vi "Handle.vi"(8 "error in (no error)":errorcluster, 10 "Error In":errorcluster, 11 "ErrorHandler(Handler) in":refnum<class "ErrorHandler(Handler).lvclass">) -> (0 "error out":errorcluster, 2 "handled?":bool, 3 "ErrorHandler(Handler) out":refnum<class "ErrorHandler(Handler).lvclass">)   [LabVIEW 2014, in "Chain Of Responsibility Pattern.lvlib" / "ErrorHandler(Handler).lvclass"]
uses:
  ErrorHandler(Handler).lvclass
  ErrorHandler(Handler).lvclass/ErrorHandler(Handler).ctl
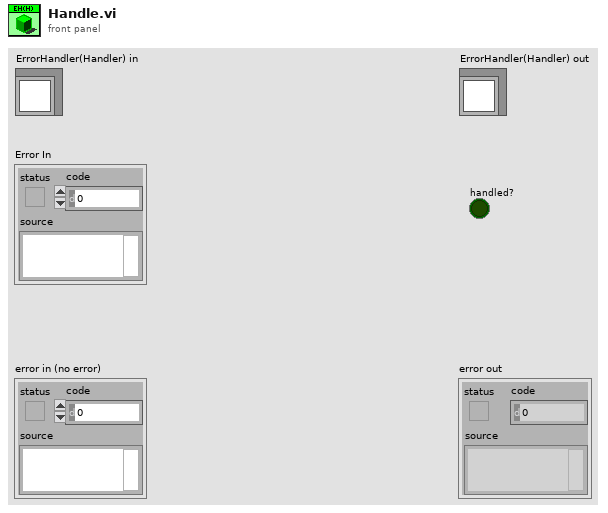
[diagram p1: front panel]
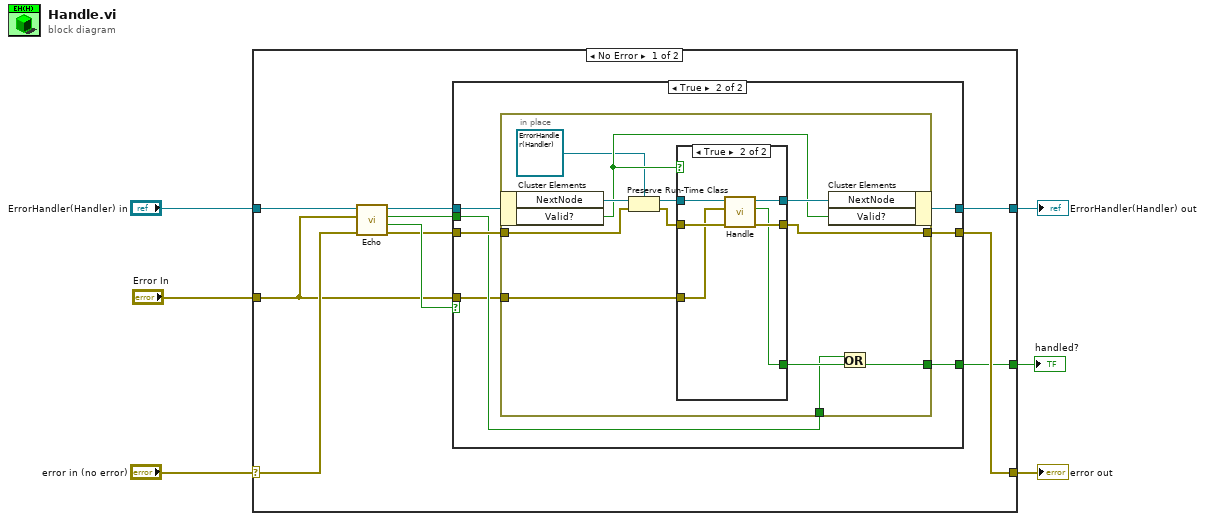
[diagram p0: block diagram]
diagram:
  n1 = case shown="No Error" "error in (no error)" {
    selector: "error in (no error)" -> [w15 w48]
    tunnel: [w10 w48] -> w5
    tunnel: [w11 w47] -> w3
    tunnel: "ErrorHandler(Handler) in" -> [w16 w47]
    tunnel: "Error In" -> [w7 _]
    tunnel: [w8 _] -> w1
    frame No Error {
      n2 = call-dynamic "Echo.vi"("error in (no error)"=w15, "Error In"=w7, "HandlerCore in"=w16) -> ("error out"=w12:errorcluster, "Still Pass?"=w14:bool, "handled?"=w9:bool, "HandlerCore out"=w13:refnum<class "ErrorHandler(Handler).lvclass">)  [unwired: 5 in]
      n3 = case shown="True" w14 {
        tunnel: w13 -> [w19 w25]
        tunnel: w12 -> [w18 w26]
        tunnel: [w19 w24] -> w11
        tunnel: [w18 w23] -> w10
        tunnel: w9 -> [w17 w21]
        tunnel: [w17 w22] -> w8
        tunnel: w7 -> [_ w20]
        frame False {
        }
        frame True {
          n4 = in-place {
            in-place-border: w26 -> [w38]
            in-place-border: [w32] -> w23
            in-place-border: [w29] -> w22
            in-place-border: w21 -> [w28]
            in-place-border: w20 -> [w27]
            n5 = in-place-cluster #1(w25) -> ("NextNode"=w36:refnum<class "HandlerCore.lvclass">, "Valid?"=w33:bool)
            n6 = Preserve Run-Time Class(object in=w36, error in=w38, 2:refnum<class "ErrorHandler(Handler).lvclass"> refnum ("ErrorHandler(Handler)")) -> (object out=w37:refnum<class "ErrorHandler(Handler).lvclass">, error out=w35:errorcluster)
            n7 = case shown="True" w33 {
              tunnel: w37 -> [w40 w46]
              tunnel: w35 -> [w39 w44]
              tunnel: [w40 w45] -> w34
              tunnel: [w39 w43] -> w32
              tunnel: [_ w42] -> w31
              tunnel: w27 -> [_ w41]
              frame False {
              }
              frame True {
                n8 = call "Handle.vi"("error in (no error)"=w44, "Error In"=w41, "ErrorHandler(Handler) in"=w46) -> ("error out"=w43:errorcluster, "handled?"=w42:bool, "ErrorHandler(Handler) out"=w45:refnum<class "ErrorHandler(Handler).lvclass">)  [unwired: 6 in]
              }
            }
            n9 = in-place-cluster #1("NextNode"=w34, "Valid?"=w33) -> (w24:refnum<class "ErrorHandler(Handler).lvclass">)
            n10 = Or(x=w28, y=w31) -> (x .or. y?=w29:bool)
          }
        }
      }
    }
    frame Error {
    }
  }
  "error out" <- w5
  "ErrorHandler(Handler) out" <- w3
  "handled?" <- w1
